vi "updateExposureTime.vi"(8 "error in (no error)":errorcluster, 10 "Pane":refnum<vi>, 11 "ICSettingsViewer in":refnum<class "ICSettingsViewer.lvclass">) -> (0 "error out":errorcluster, 2 "Pane out":refnum<vi>, 3 "ICSettingsViewer out":refnum<class "ICSettingsViewer.lvclass">)   [LabVIEW 2011, in "Views.lvlib" / "Camera.lvlib" / "ICSettingsViewer.lvclass"]
uses:
  ICSettingsViewer.lvclass
  ICSettingsViewer.lvclass/ICSettingsViewer.ctl
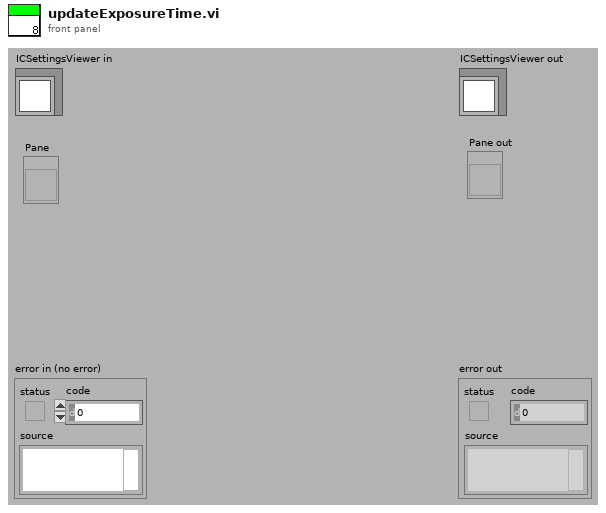
[diagram p1: front panel]
types:
  T1 = enum16{"exposure", "gain", "image_number", "Triggering", "start_trigger"}
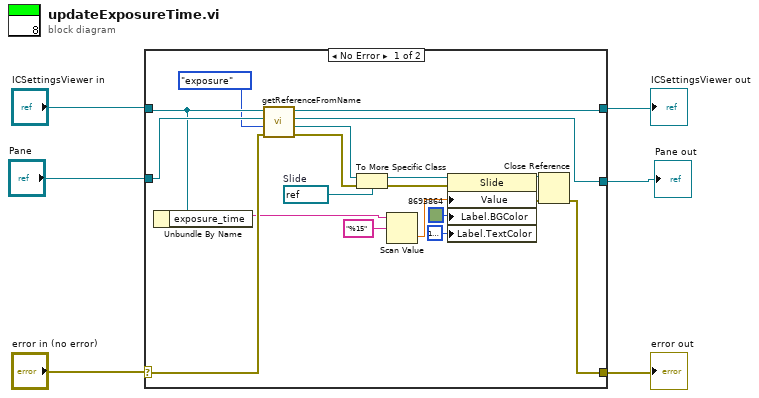
[diagram p0: block diagram]
diagram:
  n1 = case shown="No Error" "error in (no error)" {
    selector: "error in (no error)" -> [w24 w27]
    tunnel: [w12 w27] -> w2
    tunnel: [w11 w26] -> w3
    tunnel: "ICSettingsViewer in" -> [w17 w26]
    tunnel: "Pane" -> [w25 _]
    tunnel: [w23 _] -> w4
    frame No Error {
      w19 = refnum<vi> refnum  # Slide
      n2 = Unbundle By Name(w17) -> ("exposure_time"=w10:string)
      n3 = call "getReferenceFromName.vi"("error in (no error)"=w24, "referenceName"=T1."exposure", "Pane"=w25, "ICSettingsViewer in"=w17) -> ("error out"=w22:errorcluster, "Ctl Refnum"=w18:refnum<vi>, "Pane out"=w23:refnum<vi>, "ICSettingsViewer out"=w11:refnum<class "ICSettingsViewer.lvclass">)  [unwired: 3 in, 1 out]
      n4 = To More Specific Class(target class=w19, reference=w18, error in=w22) -> (specific class reference=w21:refnum<vi>, error out=w20:errorcluster)
      n5 = Scan Value(string=w10, format string="%15") -> (value=w15:dbl)  [unwired: 1 in, 1 out]
      n6 = property class="Slide"(reference=w21, error in=w20, "Value"=w15, "Label.BGColor"=u32 8693864, "Label.TextColor"=u32 16777222) -> (reference out=w14:refnum<vi>, error out=w13:errorcluster)
      n7 = Close Reference(reference=w14, error in (no error)=w13) -> (error out=w12:errorcluster)
    }
    frame Error {
    }
  }
  "error out" <- w2
  "ICSettingsViewer out" <- w3
  "Pane out" <- w4
